vi "GetAcPwrBdcstEvents.vi"(7 "error in (no error)":errorcluster) -> (3 "Event Registration Refnum":T1, 5 "error out":errorcluster)   [LabVIEW 2018, in "Test.lvclass"]
uses:
  Test.lvclass
  Typedef/AcPwrEventReg.ctl
  AcPwr/AcPwrModule/Protected/clEventType.ctl
  AcPwr/AcPwrModule/AcPwrModule.lvlib
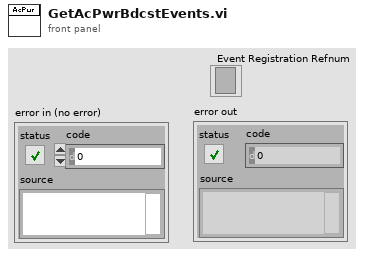
[diagram p1: front panel]
types:
  T1 = typedef "Test.lvclass/AcPwrEventReg.ctl" = refnum<event-registration>
  T2 = typedef "AcPwrModule.lvlib/clBroadcastEvents.ctl" = cluster{"DidInit":refnum<user-event>, "StatusUpdate":refnum<user-event>, "ErrorReport":refnum<user-event>, "DidStop":refnum<user-event>, "PathToINI":refnum<user-event>, "Measurements":refnum<user-event>, "LoadConfigFile":refnum<user-event>, "GetSettings":refnum<user-event>, "SetSettings":refnum<user-event>, "GetType&ID":refnum<user-event>, "GotSettings":refnum<user-event>}
  T3 = cluster{"Measurements":refnum<user-event>, "ErrorReport":refnum<user-event>, "GetSettings":refnum<user-event>, "SetSettings":refnum<user-event>, "GotSettings":refnum<user-event>}
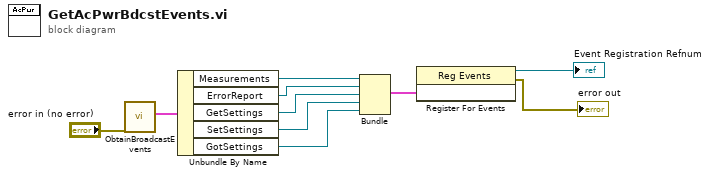
[diagram p0: block diagram]
diagram:
  n1 = call "ObtainBroadcastEvents.vi"("error in (no error)"="error in (no error)") -> ("clAcPwrEvents"=w7:T2)  [unwired: 9 in, 1 out]
  n2 = Unbundle By Name(w7) -> ("Measurements"=w10:refnum<user-event>, "ErrorReport"=w8:refnum<user-event>, "GetSettings"=w6:refnum<user-event>, "SetSettings"=w5:refnum<user-event>, "GotSettings"=w2:refnum<user-event>)
  n3 = Bundle("Measurements"=w10, "ErrorReport"=w8, "GetSettings"=w6, "SetSettings"=w5, "GotSettings"=w2) -> (w9:T3)  [unwired: 1 in]
  n4 = register-events(w9) -> (reference out=→"Event Registration Refnum":refnum<event-registration>, error out=→"error out":errorcluster)  [unwired: 2 in]
